vi "Large int-add a and b.vi"(8 "error in (no error)":errorcluster, 10 "b = Large int (decimal)":string, 11 "a = Large int (decimal)":string) -> (0 "error out":errorcluster, 2 "T = the inputs are valid integers":bool, 3 "c = a x b":string)   [LabVIEW 2021, in "Numeric Utilities.lvlib"]
uses:
  Numeric Utilities.lvlib
panel:
  out "shorter integer (with prefix)":string
  out "longer integer":string
  out "shorter integer":string
  out "Loop iteration":i32
  # "Development\ncontrols/indicators useful for development and testing, but which are not outputs of the VI"
  # "Input\nInputs to the VI"
  # "Output\nOutputs of the VI"
  # "Description\n\nBlank VI with error handling case. \n\nSummarize the use of this VI in this space."
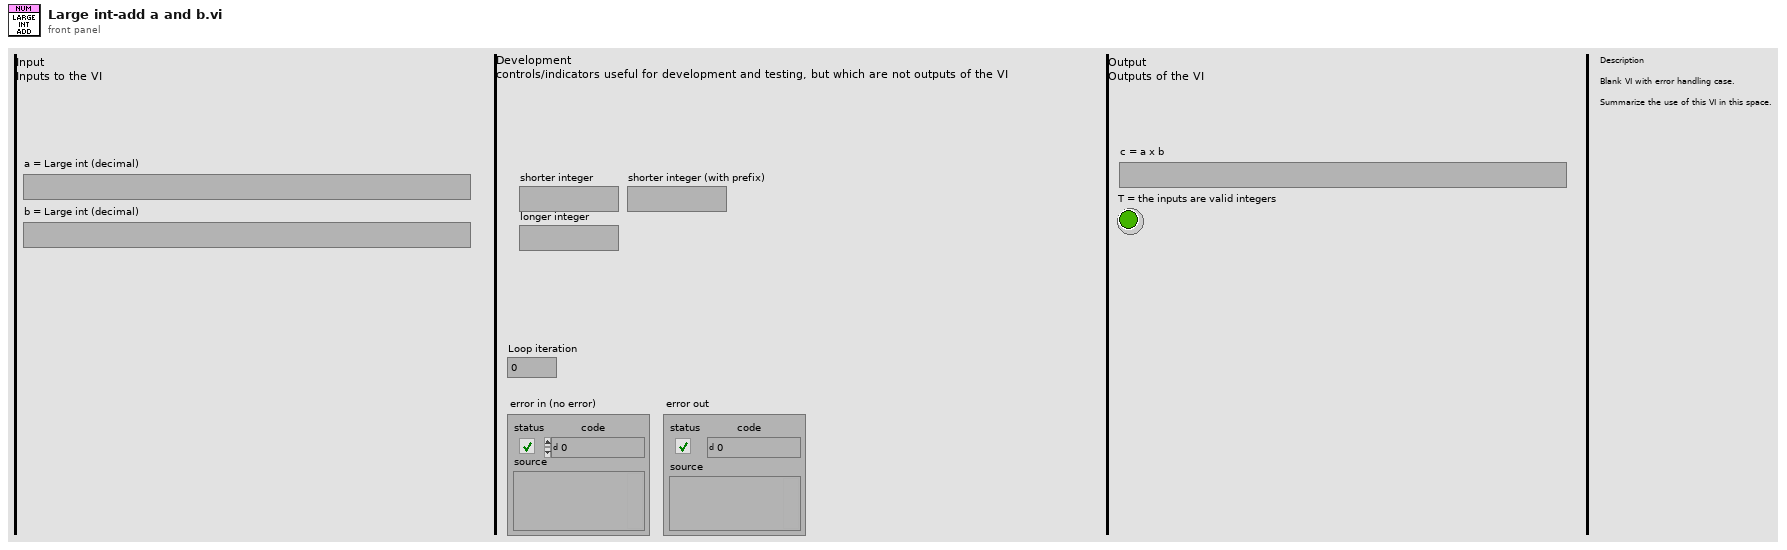
[diagram p1: front panel]
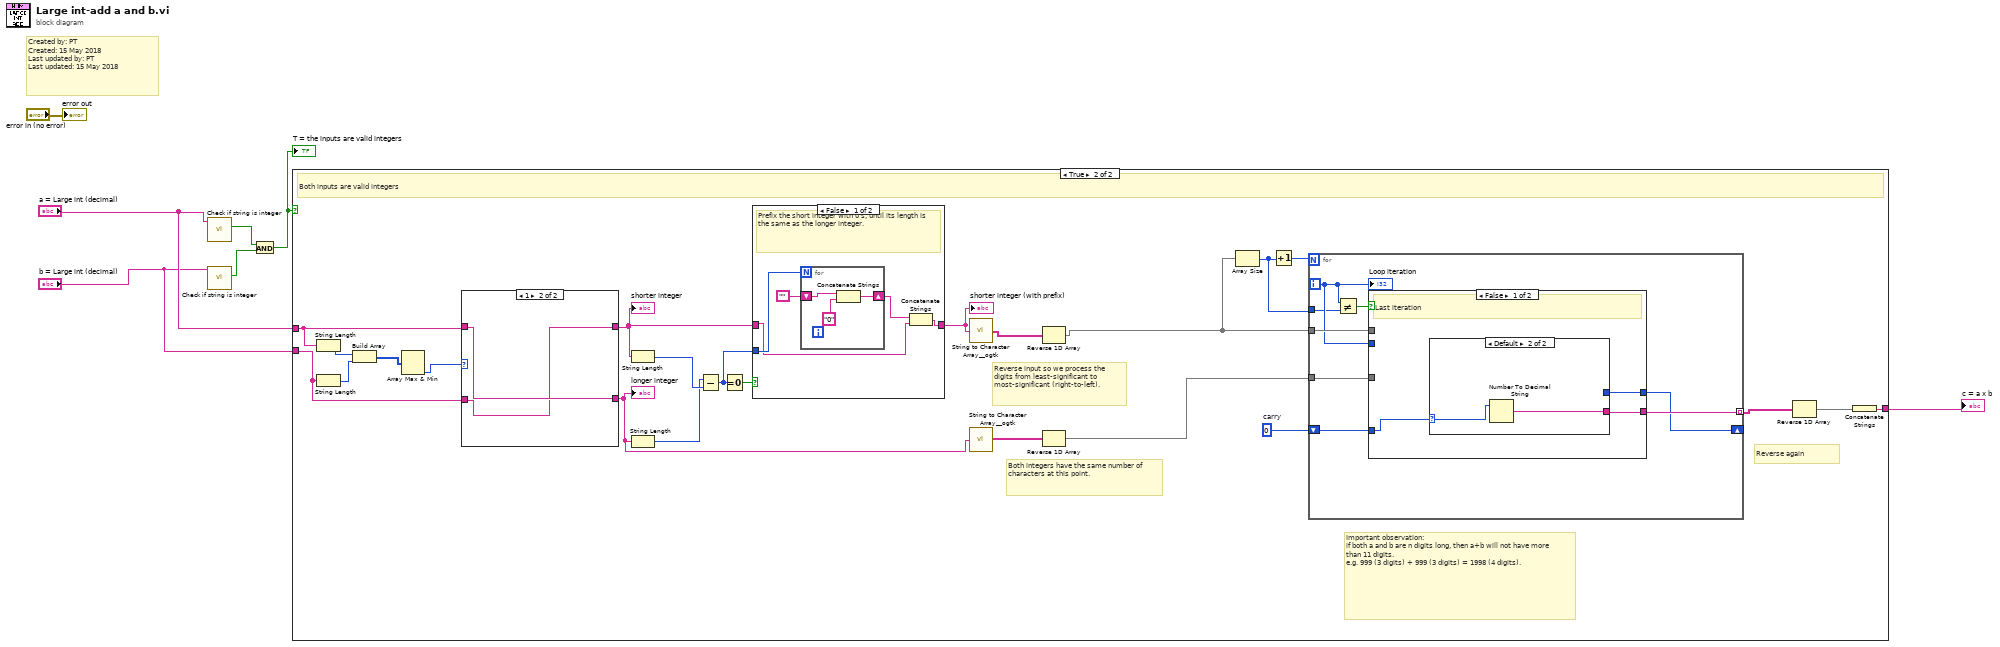
[diagram p0: block diagram]
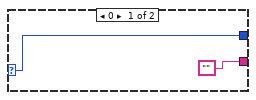
[diagram p5: hidden frame]
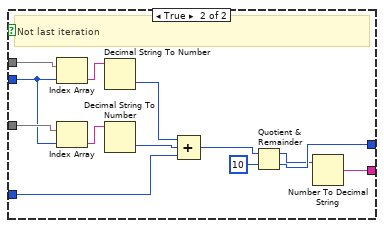
[diagram p6: hidden frame]
diagram:
  # "Created by: PT\nCreated: 15 May 2018\nLast updated by: PT\nLast updated: 15 May 2018"
  n1 = call "Check if string is integer.vi"("string in"="a = Large int (decimal)") -> ("T = string contains an integer"=w5:bool)  [unwired: 8 in, 2 out]
  n2 = call "Check if string is integer.vi"("string in"="b = Large int (decimal)") -> ("T = string contains an integer"=w4:bool)  [unwired: 8 in, 2 out]
  n3 = And(x=w5, y=w4) -> (x .and. y?=w3:bool)
  "T = the inputs are valid integers" <- w3
  n4 = case shown="True" w3 {
    tunnel: "a = Large int (decimal)" -> [_ w10]
    tunnel: [_ w29] -> w6
    tunnel: "b = Large int (decimal)" -> [_ w9]
    frame False {
      # "Input is not a number"
    }
    frame True {
      w30 = 0  # carry
      # "Both integers have the same number of characters at this point."
      # "Important observation:\nif both a and b are n digits long, then a+b will not have more than 11 digits.\ne.g. 999 (3 digits) + 999 (3 digits) = 1998 (4 digits)."
      # "Reverse again"
      # "Reverse input so we process the digits from least-significant to most-significant (right-to-left)."
      # "Both inputs are valid integers"
      n5 = String Length(string=w10) -> (length=w28:i32)
      n6 = String Length(string=w9) -> (length=w27:i32)
      n7 = Build Array(w28, w27) -> (w26:i32[])
      n8 = Array Max & Min(array=w26) -> (min index (indices)=w8:i32)  [unwired: 3 out]
      n9 = case shown="1" w8 {
        tunnel: w10 -> [w41 w43]
        tunnel: [w41 w42] -> w23
        tunnel: [w40 w43] -> w19
        tunnel: w9 -> [w40 w42]
        frame 0, Default {
        }
        frame 1 {
        }
      }
      "shorter integer" <- w23
      "longer integer" <- w19
      n10 = String Length(string=w23) -> (length=w25:i32)
      n11 = String Length(string=w19) -> (length=w24:i32)
      n12 = Subtract(x=w24, y=w25) -> (x-y=w21:i32)
      n13 = Equal To 0?(x=w21) -> (x = 0?=w22:bool)
      n14 = case shown="False" w22 {
        tunnel: w23 -> [w32 w39]
        tunnel: w21 -> [w34 _]
        tunnel: [w31 w39] -> w20
        frame False {
          # "Prefix the short integer with 0's, until its length is the same as the longer integer."
          n15 = for {
            N: w34 -> [_]
            shift-right: [w36] -> w33
            shift-left: "" -> [w38]
            n16 = Concatenate Strings(w38, "0") -> (w36:string)
          }
          n17 = Concatenate Strings(w33, w32) -> (w31:string)
        }
        frame True {
          # "The \"short\" integer and the \"long\" integer have the same length. No need to prefix the short integer with 0's."
        }
      }
      "shorter integer (with prefix)" <- w20
      n18 = call <userlib>:"String to Character Array__ogtk.vi"("Input String"=w20) -> ("Character Array"=w18:string[])
      n19 = call <userlib>:"String to Character Array__ogtk.vi"("Input String"=w19) -> ("Character Array"=w17:string[])
      n20 = Reverse 1D Array(array=w18) -> (reversed array=w13:string[])
      n21 = Reverse 1D Array(array=w17) -> (reversed array=w16:string[])
      n22 = Array Size(array=w13) -> (size(s)=w11:i32)
      n23 = Increment(x=w11) -> (x+1=w12:i32)
      n24 = for {
        N: w12 -> [_]
        tunnel: w13 -> [w48]
        shift-right: [w49] -> _
        shift-left: w30 -> [w51]
        tunnel: [w50] -> w15 mode=indexing
        tunnel: w16 -> [w47]
        tunnel: w11 -> [w45]
        i -> [w46]
        n25 = Not Equal?(x=w46, y=w45) -> (x != y?=w44:bool)
        n26 = case shown="False" w44 {
          tunnel: w51 -> [w54 w71]
          tunnel: [w53 w70] -> w50
          tunnel: [w52 w69] -> w49
          tunnel: w48 -> [_ w63]
          tunnel: w47 -> [_ w61]
          tunnel: w46 -> [_ w59]
          frame False {
            # "Last iteration"
            n27 = case shown="Default" w54 {
              selector: w54 -> [w55 w58]
              tunnel: ["" w57] -> w53
              tunnel: [w55 _] -> w52
              frame 0 {
              }
              frame Default {
                n28 = Number To Decimal String(number=w58) -> (decimal integer string=w57:string)  [unwired: 1 in]
              }
            }
          }
          frame True {
            # "Not last iteration"
            n29 = Index Array(array=w63, index=w59) -> (element=w62:string)
            n30 = Index Array(array=w61, index=w59) -> (element=w60:string)
            n31 = Decimal String To Number(string=w62) -> (number=w65:i32)  [unwired: 2 in, 1 out]
            n32 = Decimal String To Number(string=w60) -> (number=w64:i32)  [unwired: 2 in, 1 out]
            n33 = Compound Arithmetic op=ADD(w65, w64, w71) -> (w68:i32)
            n34 = Quotient & Remainder(x=w68, y=10) -> (x-y*floor(x/y)=w66:i32, floor(x/y)=w69:i32)
            n35 = Number To Decimal String(number=w66) -> (decimal integer string=w70:string)  [unwired: 1 in]
          }
        }
        "Loop iteration" <- w46
      }
      n36 = Reverse 1D Array(array=w15) -> (reversed array=w14:string[])
      n37 = Concatenate Strings(w14) -> (w29:string)
    }
  }
  "c = a x b" <- w6
  "error out" <- "error in (no error)"
